vi "Write indent.vi"(10 "indent":i32, 11 "MsgSerializer in":refnum<class "MsgSerializer.JSON.lvclass">) -> (3 "MsgSerializer out":refnum<class "MsgSerializer.JSON.lvclass">)   [LabVIEW 2013]
uses:
  MsgSerializer.JSON.lvclass
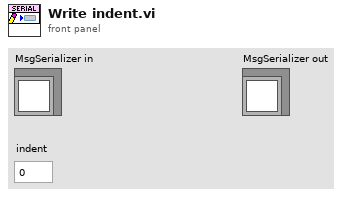
[diagram p1: front panel]
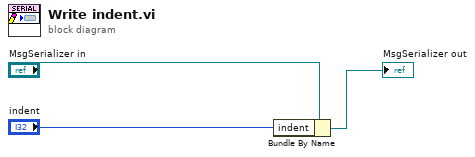
[diagram p0: block diagram]
diagram:
  n1 = Bundle By Name(cluster="MsgSerializer in", "indent"="indent") -> (→"MsgSerializer out":refnum<class "MsgSerializer.JSON.lvclass">)
